vi "Chrg_Dschrg_nodaq_nocrio.vi"(0 "Output Safety":T1, 3 "PS type":enum16{"NHR", "ITECH"}(ring), 4 "PS VISA in":refnum<visa-resource-name>, 5 "PS error in":errorcluster caption="PS error in (no error)", 6 "CyclePath":path=path "C:/Users/ga11/Desktop/VI/results/3PtestCharge.lvm" caption="Filename", 7 "Battery Type":T2(ring), 8 "Charge/discharge":enum8{"Charge", "Discharge"}(ring), 9 "Charge/Discharge Voltage Setpoint":dbl format="%#.6g", 11 "Current Setpoint":dbl format="%#.6g", 13 "Current Cutoff":dbl) -> (14 "PS VISA out":refnum<visa-resource-name>, 19 "PS error out":errorcluster)   [LabVIEW 2020]
uses:
  Drivers-NHR-9200/NHR/Public/Data/Read (Ave Current).vi
  Drivers-NHR-9200/NHR/Public/Data/Low Level/Fetch (Ave Voltage).vi
  Drivers-Essentials/NH Research Regenerative Test Series.lvlib
  Drivers-IT-M3400/IT-M3400.lvlib
panel:
  out "Read Ave Current (A)":dbl
  out "Read Ave Voltage (V)":dbl
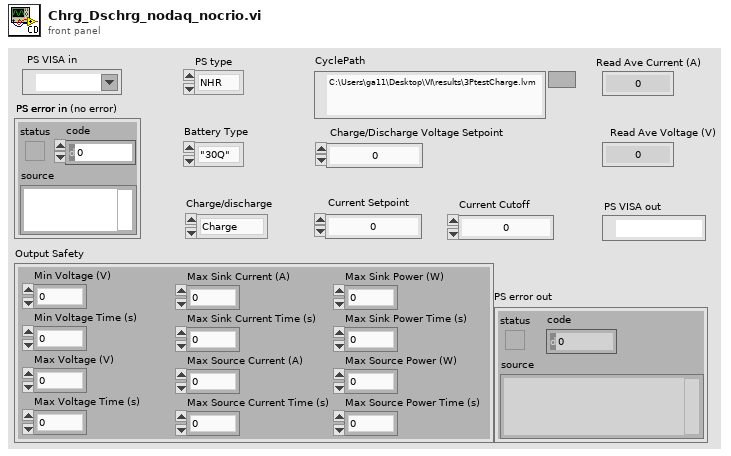
[diagram p1: front panel]
types:
  T1 = cluster{"Min Voltage (V)":dbl, "Min Voltage Time (s)":dbl, "Max Voltage (V)":dbl, "Max Voltage Time (s)":dbl, "Max Sink Current (A)":dbl, "Max Sink Current Time (s)":dbl, "Max Source Current (A)":dbl, "Max Source Current Time (s)":dbl, "Max Sink Power (W)":dbl, "Max Sink Power Time (s)":dbl, "Max Source Power (W)":dbl, "Max Source Power Time (s)":dbl}
  T2 = enum16{"\"30Q\"", "\"40T\"", "\"2P30Q\"", "\"3P30Q\"", "\"Nissan Leaf\""}
  T3 = cluster{"Voltage Enabled":bool, "Current Enabled":bool, "Power Enabled":bool, "Resistance Enabled":bool}
  T4 = cluster{"Baud Rate":u32, "Parity":u16, "Data Bits":u16, "Stop Bits":u16, "Flow Control":u16}
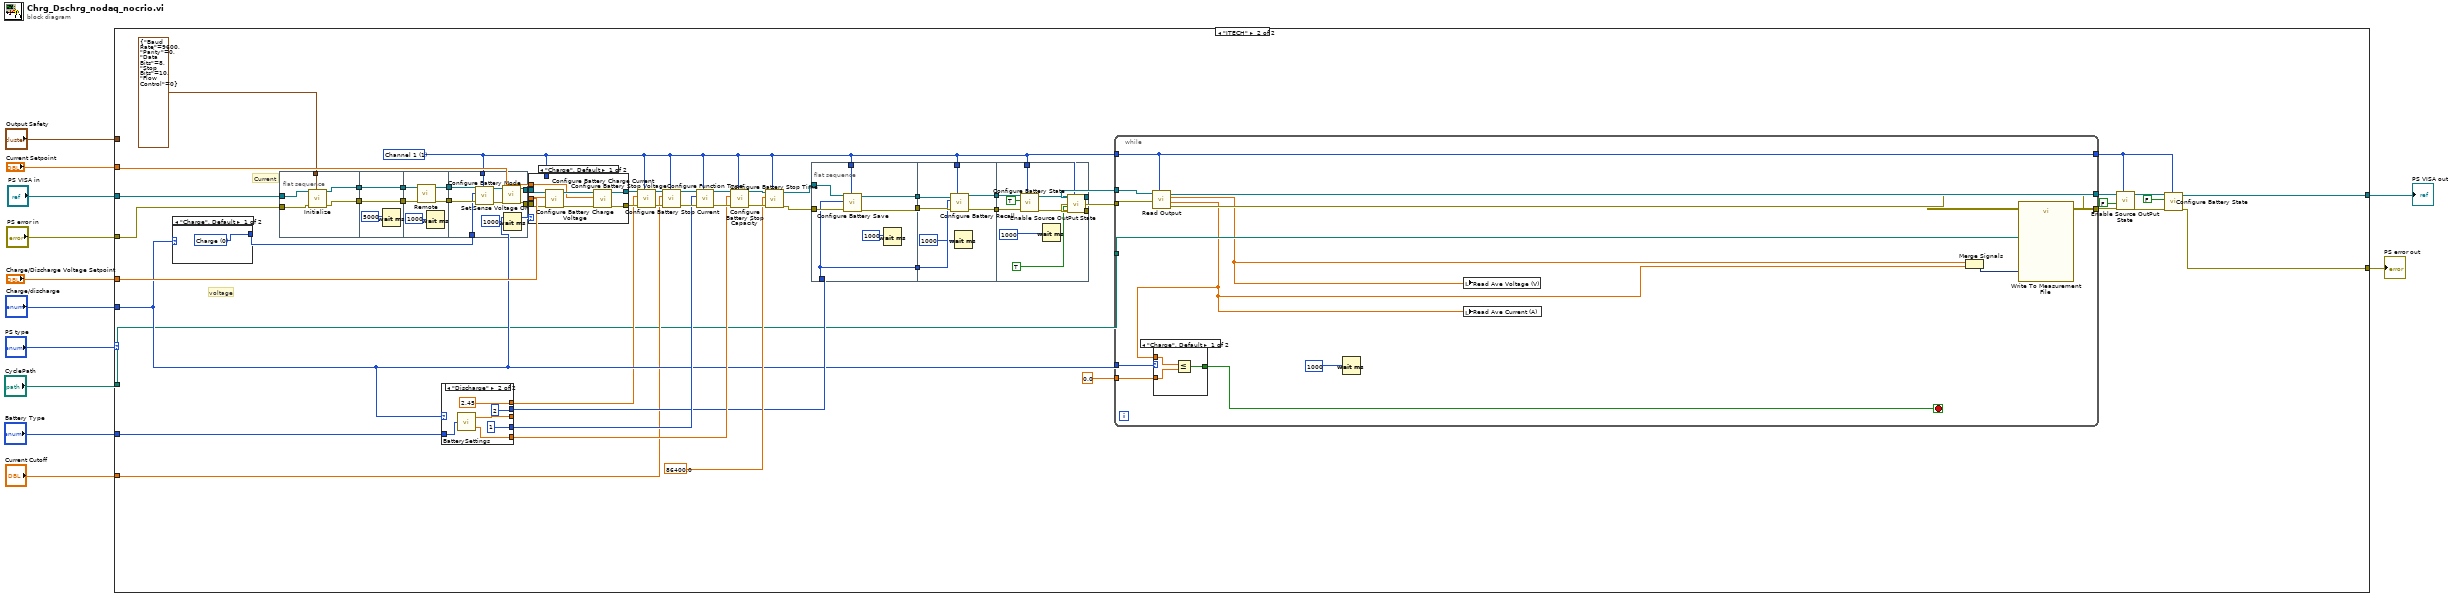
[diagram p0: block diagram]
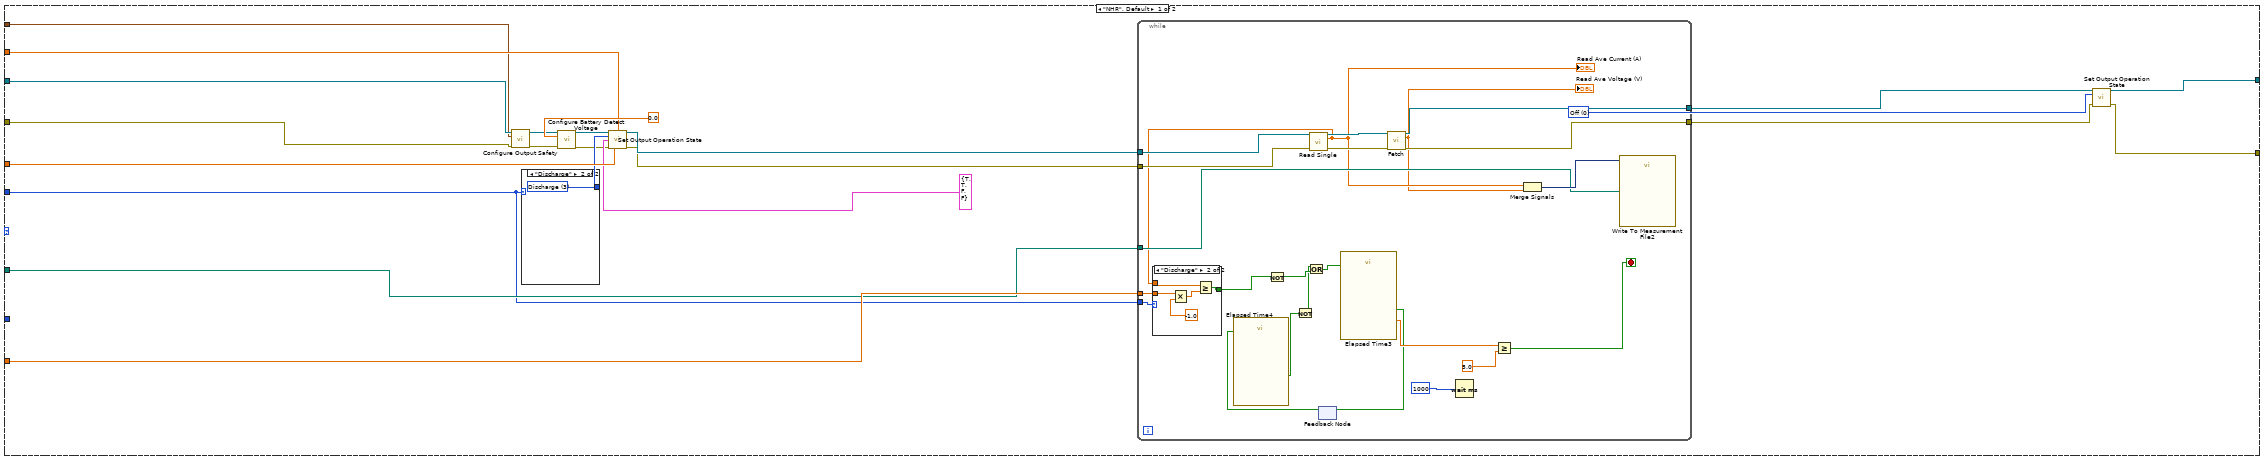
[diagram p2: hidden frame]
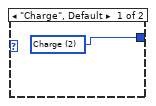
[diagram p3: hidden frame]
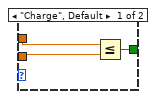
[diagram p4: hidden frame]
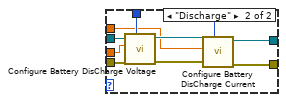
[diagram p5: hidden frame]
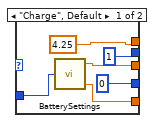
[diagram p6: hidden frame]
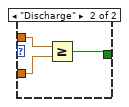
[diagram p7: hidden frame]
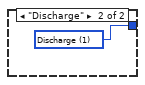
[diagram p8: hidden frame]
diagram:
  n1 = case shown="\"ITECH\"" "PS type" {
    tunnel: "Charge/Discharge Voltage Setpoint" -> [w34 w105]
    tunnel: "Current Setpoint" -> [w18 w103]
    tunnel: "Current Cutoff" -> [w31 w73]
    tunnel: "CyclePath" -> [w28 w71]
    tunnel: "PS VISA in" -> [w14 w84]
    tunnel: "PS error in" -> [w15 w83]
    tunnel: [w23 w70] -> w2
    tunnel: [w22 w104] -> w6
    tunnel: "Charge/discharge" -> [w19 w74]
    tunnel: "Battery Type" -> [_ w102]
    tunnel: "Output Safety" -> [w13 _]
    frame "NHR", Default {
      w27 = 0 items=["Off", "Standby", "Charge", "Discharge", "Battery"] ("Mode (0: Off)")
      n2 = call "Configure Output Safety.vi"("VISA resource name"=w14, "Output Safety"=w13, "error in (no error)"=w15) -> ("VISA resource name out"=w16:refnum<visa-resource-name>, "error out"=w17:errorcluster)  [unwired: 11 in]
      n3 = case shown="\"Discharge\"" w19 {
        tunnel: [w35 w36] -> w29
        frame "Charge", Default {
          w35 = 2 items=["Off", "Standby", "Charge", "Discharge", "Battery"] ("Mode (0: Off)")
        }
        frame "Discharge" {
          w36 = 3 items=["Off", "Standby", "Charge", "Discharge", "Battery"] ("Mode (0: Off)")
        }
      }
      n4 = call "Configure Battery Detect Voltage.vi"("VISA resource name"=w16, "Battery Detect Voltage (0V)"=0.0, "error in (no error)"=w17) -> ("VISA resource name out"=w26:refnum<visa-resource-name>, "error out"=w25:errorcluster)  [unwired: 11 in]
      n5 = call "Set Output Operation State.vi"("VISA resource name"=w26, "Voltage Setpoint (0 V)"=w34, "Current Setpoint (0 A)"=w18, "Mode (0: Off)"=w29, "Enable"=T3 {"Voltage Enabled"=TRUE, "Current Enabled"=TRUE, "Power Enabled"=FALSE, "Resistance Enabled"=FALSE}, "error in (no error)"=w25) -> ("VISA resource name out"=w33:refnum<visa-resource-name>, "error out"=w32:errorcluster)  [unwired: 8 in]
      n6 = while {
        tunnel: w33 -> [w57]
        tunnel: w32 -> [w56]
        tunnel: w31 -> [w41]
        tunnel: w28 -> [w44]
        tunnel: [w43] -> w21
        tunnel: [w42] -> w20
        tunnel: w19 -> [w40]
        stop <- w47 stop-if-true
        n7 = call-poly "Read Single.vi"("VISA resource name"=w57, "error in (no error)"=w56) -> ("VISA resource name out"=w58:refnum<visa-resource-name>, "Ave Current (A)"=w39:dbl, "error out"=w59:errorcluster)  [unwired: 11 in]
        "Read Ave Current (A)" <- w39
        n8 = case shown="\"Discharge\"" w40 {
          tunnel: w41 -> [w61 w66]
          tunnel: w39 -> [w62 w64]
          tunnel: [w60 w63] -> w38
          frame "Charge", Default {
            n9 = Less Or Equal?(x=w62, y=w61) -> (x <= y?=w60:bool)
          }
          frame "Discharge" {
            n10 = Multiply(x=w66, y=-1.0) -> (x*y=w65:dbl)
            n11 = Greater Or Equal?(x=w64, y=w65) -> (x >= y?=w63:bool)
          }
        }
        n12 = Not(x=w38) -> (.not. x?=w53:bool)
        n13 = feedback #1() -> (w45:bool)  [unwired: 1 in]
        n14 = call "Elapsed Time4"("Reset"=w45) -> ("Time has Elapsed"=w52:bool)  [unwired: 11 in, 7 out]
        n15 = Not(x=w52) -> (.not. x?=w51:bool)
        n16 = Or(x=w51, y=w53) -> (x .or. y?=w50:bool)
        n17 = call "Elapsed Time3"("Reset"=w50) -> ("Elapsed Time (s)"=w49:dbl, "Time has Elapsed"=w46:bool)  [unwired: 11 in, 6 out]
        n18 = feedback-in #1(w46) -> ()
        n19 = call-poly "Fetch.vi"("VISA resource name"=w58, "error in (no error)"=w59) -> ("VISA resource name out"=w43:refnum<visa-resource-name>, "Ave Voltage (V)"=w37:dbl, "error out"=w42:errorcluster)  [unwired: 11 in]
        "Read Ave Voltage (V)" <- w37
        n20 = Wait (ms)(milliseconds to wait=1000) -> ()  [unwired: 1 out]
        n21 = Greater Or Equal?(x=w49, y=5.0) -> (x >= y?=w47:bool)
        n22 = Merge Signals "Merge Signals"(w39, w37) -> (w55:dynamicdata)
        n23 = call "Write To Measurement File2"("Signals"=w55, "Filename"=w44) -> ()  [unwired: 15 in, 3 out]
      }
      n24 = call "Set Output Operation State.vi"("VISA resource name"=w21, "Mode (0: Off)"=w27, "error in (no error)"=w20) -> ("VISA resource name out"=w23:refnum<visa-resource-name>, "error out"=w22:errorcluster)  [unwired: 11 in]
    }
    frame "ITECH" {
      w76 = 1 items=["Channel 1"=1, "Channel 2"=2, "Channel 3"=3, "Channel 4"=4, "Channel 5"=5, "Channel 6"=6, "Channel 7"=7, "Channel 8"=8, "Channel 8"=9, "Channel 10"=10, "Channel 11"=11, "Channel 12"=12, "Channel 13"=13, "Channel 14"=14, "Channel 15"=15, "Channel 16"=16] ("Channel")
      # "voltage"
      # "Current"
      n25 = case shown="\"Charge\", Default" w74 {
        tunnel: [w215 w216] -> w90
        frame "Charge", Default {
          w215 = u8 0 items=["Charge", "Discharge"] ("Battery Mode")
        }
        frame "Discharge" {
          w216 = u8 1 items=["Charge", "Discharge"] ("Battery Mode")
        }
      }
      n26 = flat-sequence {
        tunnel: [w121] -> w88
        tunnel: [w122] -> w86
        tunnel: T4 {"Baud Rate"=9600, "Parity"=0, "Data Bits"=8, "Stop Bits"=10, "Flow Control"=0} ("Serial Configuration") -> [w125]
        tunnel: w83 -> [w124]
        tunnel: w84 -> [w123]
        tunnel: w88 -> [w128]
        tunnel: [w128] -> w87
        tunnel: w86 -> [w127]
        tunnel: [w127] -> w85
        tunnel: [w133] -> w92
        tunnel: [w132] -> w91
        tunnel: w87 -> [w131]
        tunnel: w85 -> [w130]
        tunnel: w92 -> [w139]
        tunnel: w91 -> [w141]
        tunnel: w76 -> [w142]
        tunnel: w90 -> [w140]
        tunnel: [w135] -> w69
        tunnel: [w134] -> w68
        frame #0 {
          n27 = call "Initialize.vi"("Serial Configuration"=w125, "error in"=w124, "VISA resource name"=w123) -> ("error out"=w122:errorcluster, "VISA resource name out"=w121:refnum<visa-resource-name>)  [unwired: 7 in]
        }
        frame #1 {
          n28 = Wait (ms)(milliseconds to wait=5000) -> ()  [unwired: 1 out]
        }
        frame #2 {
          n29 = call "Remote.vi"("error in"=w130, "VISA resource name"=w131) -> ("error out"=w132:errorcluster, "VISA resource name out"=w133:refnum<visa-resource-name>)  [unwired: 8 in]
          n30 = Wait (ms)(milliseconds to wait=1000) -> ()  [unwired: 1 out]
        }
        frame #3 {
          n31 = call "Configure Battery Mode.vi"("Channel"=w142, "error in"=w141, "Battery Mode"=w140, "VISA resource name"=w139) -> ("error out"=w136:errorcluster, "VISA resource name out"=w137:refnum<visa-resource-name>)  [unwired: 6 in]
          n32 = call "Set Sense Voltage On.vi"("error in"=w136, "VISA resource name"=w137) -> ("error out"=w135:errorcluster, "VISA resource name out"=w134:refnum<visa-resource-name>)  [unwired: 8 in]
          n33 = Wait (ms)(milliseconds to wait=1000) -> ()  [unwired: 1 out]
        }
      }
      n34 = case shown="\"Discharge\"" w74 {
        tunnel: w102 -> [w189 w195]
        tunnel: [w188 w193] -> _
        tunnel: [u8 0 ("File") u8 1 ("File")] -> w78
        tunnel: [u8 1 ("File") u8 2 ("File")] -> w75
        tunnel: [w185 w191] -> w77
        tunnel: [4.25 2.45] -> w72
        frame "Charge", Default {
          n35 = call "BatterySettings.vi"("Battery Type"=w189) -> ("RatedCapacity (Ah)"=w185:dbl, "Max Voltage (V)"=w188:dbl)  [unwired: 2 in, 1 out]
        }
        frame "Discharge" {
          n36 = call "BatterySettings.vi"("Battery Type"=w195) -> ("RatedCapacity (Ah)"=w191:dbl, "Min Voltage (V)"=w193:dbl)  [unwired: 2 in, 1 out]
        }
      }
      n37 = case shown="\"Charge\", Default" w74 {
        tunnel: w68 -> [w174 w183]
        tunnel: w69 -> [w173 w182]
        tunnel: [w168 w179] -> w112
        tunnel: [w167 w178] -> w111
        tunnel: w76 -> [_ w177]
        tunnel: w105 -> [w170 w176]
        tunnel: w103 -> [w169 w175]
        frame "Charge", Default {
          n38 = call "Configure Battery Charge Voltage.vi"("error in"=w173, "Charge Voltage(V)"=w170, "VISA resource name"=w174) -> ("error out"=w171:errorcluster, "VISA resource name out"=w172:refnum<visa-resource-name>)  [unwired: 6 in]
          n39 = call "Configure Battery Charge Current.vi"("error in"=w171, "Charge Current(A)"=w169, "VISA resource name"=w172) -> ("error out"=w167:errorcluster, "VISA resource name out"=w168:refnum<visa-resource-name>)  [unwired: 7 in]
        }
        frame "Discharge" {
          n40 = call "Configure Battery DisCharge Voltage.vi"("Channel"=w177, "error in"=w182, "Discharge Voltage(V)"=w176, "VISA resource name"=w183) -> ("error out"=w180:errorcluster, "VISA resource name out"=w181:refnum<visa-resource-name>)  [unwired: 6 in]
          n41 = call "Configure Battery DisCharge Current.vi"("Channel"=w177, "error in"=w180, "Discharge Current(A)"=w175, "VISA resource name"=w181) -> ("error out"=w178:errorcluster, "VISA resource name out"=w179:refnum<visa-resource-name>)  [unwired: 6 in]
        }
      }
      n42 = call "Configure Battery Stop Voltage.vi"("Channel"=w76, "error in"=w111, "Stop Voltage(V)"=w72, "VISA resource name"=w112) -> ("error out"=w119:errorcluster, "VISA resource name out"=w120:refnum<visa-resource-name>)  [unwired: 6 in]
      n43 = call "Configure Battery Stop Current.vi"("Channel"=w76, "error in"=w119, "Stop Current(A)"=w73, "VISA resource name"=w120) -> ("error out"=w80:errorcluster, "VISA resource name out"=w82:refnum<visa-resource-name>)  [unwired: 6 in]
      n44 = call "Configure Function Type.vi"("Channel"=w76, "error in"=w80, "Function Type"=w78, "VISA resource name"=w82) -> ("error out"=w79:errorcluster, "VISA resource name out"=w81:refnum<visa-resource-name>)  [unwired: 6 in]
      n45 = call "Configure Battery Stop Capacity.vi"("Channel"=w76, "error in"=w79, "Stop Capacity(Ah)"=w77, "VISA resource name"=w81) -> ("error out"=w117:errorcluster, "VISA resource name out"=w118:refnum<visa-resource-name>)  [unwired: 6 in]
      n46 = call "Configure Battery Stop Time.vi"("Channel"=w76, "error in"=w117, "Stop Time(S)"=86400.0, "VISA resource name"=w118) -> ("error out"=w94:errorcluster, "VISA resource name out"=w93:refnum<visa-resource-name>)  [unwired: 6 in]
      n47 = flat-sequence {
        tunnel: w75 -> [w148]
        tunnel: w76 -> [w143]
        tunnel: [w146] -> w97
        tunnel: [w148] -> w96
        tunnel: [w145] -> w95
        tunnel: w94 -> [w149]
        tunnel: w93 -> [w147]
        tunnel: [w152] -> w99
        tunnel: [w153] -> w98
        tunnel: w97 -> [w156]
        tunnel: w96 -> [w155]
        tunnel: w95 -> [w154]
        tunnel: w76 -> [w150]
        tunnel: [w160] -> w110
        tunnel: [w159] -> w109
        tunnel: w76 -> [w158]
        tunnel: w99 -> [w166]
        tunnel: w98 -> [w165]
        frame #0 {
          n48 = call "Configure Battery Save.vi"("Channel"=w143, "error in"=w149, "File"=w148, "VISA resource name"=w147) -> ("error out"=w146:errorcluster, "VISA resource name out"=w145:refnum<visa-resource-name>)  [unwired: 6 in]
          n49 = Wait (ms)(milliseconds to wait=1000) -> ()  [unwired: 1 out]
        }
        frame #1 {
          n50 = call "Configure Battery Recall.vi"("Channel"=w150, "error in"=w156, "File"=w155, "VISA resource name"=w154) -> ("error out"=w153:errorcluster, "VISA resource name out"=w152:refnum<visa-resource-name>)  [unwired: 6 in]
          n51 = Wait (ms)(milliseconds to wait=1000) -> ()  [unwired: 1 out]
        }
        frame #2 {
          n52 = call "Configure Battery State.vi"("Channel"=w158, "error in"=w165, "State"=TRUE, "VISA resource name"=w166) -> ("error out"=w163:errorcluster, "VISA resource name out"=w164:refnum<visa-resource-name>)  [unwired: 6 in]
          n53 = Wait (ms)(milliseconds to wait=1000) -> ()  [unwired: 1 out]
          n54 = call "Enable Source OutPut State.vi"("Channel"=w158, "error in"=w163, "State"=TRUE ("Enable Output|Intput"), "VISA resource name"=w164) -> ("error out"=w159:errorcluster, "VISA resource name out"=w160:refnum<visa-resource-name>)  [unwired: 6 in]
        }
      }
      n55 = while {
        tunnel: [w200] -> w108
        tunnel: [w198] -> w107
        tunnel: w110 -> [w208]
        tunnel: w109 -> [w207]
        tunnel: w76 -> [w199]
        tunnel: [w199] -> w106
        tunnel: w71 -> [w205]
        tunnel: 0.0 -> [w203]
        tunnel: w74 -> [w201]
        stop <- w202 stop-if-true
        n56 = call "Read Output.vi"("Channel"=w199, "error in"=w207, "VISA resource name"=w208) -> ("error out"=w198:errorcluster, "Read Current(A)"=w196:dbl, "Read Voltage(V)"=w197:dbl, "VISA resource name out"=w200:refnum<visa-resource-name>)  [unwired: 5 in]
        n57 = case shown="\"Charge\", Default" w201 {
          tunnel: w203 -> [w210 w213]
          tunnel: w196 -> [w211 w214]
          tunnel: [w209 w212] -> w202
          frame "Charge", Default {
            n58 = Less Or Equal?(x=w211, y=w210) -> (x <= y?=w209:bool)
          }
          frame "Discharge" {
            n59 = Greater Or Equal?(x=w214, y=w213) -> (x >= y?=w212:bool)
          }
        }
        n60 = Wait (ms)(milliseconds to wait=1000) -> ()  [unwired: 1 out]
        n61 = local write "Read Ave Voltage (V)"(w197) -> ()
        n62 = local write "Read Ave Current (A)"(w196) -> ()
        n63 = Merge Signals "Merge Signals"(w197, w196) -> (w206:dynamicdata)
        n64 = call "Write To Measurement File"("Signals"=w206, "Filename"=w205) -> ()  [unwired: 15 in, 3 out]
      }
      n65 = call "Enable Source OutPut State.vi"("Channel"=w106, "error in"=w107, "State"=FALSE, "VISA resource name"=w108) -> ("error out"=w115:errorcluster, "VISA resource name out"=w116:refnum<visa-resource-name>)  [unwired: 6 in]
      n66 = call "Configure Battery State.vi"("Channel"=w106, "error in"=w115, "State"=FALSE, "VISA resource name"=w116) -> ("error out"=w104:errorcluster, "VISA resource name out"=w70:refnum<visa-resource-name>)  [unwired: 6 in]
    }
  }
  "PS error out" <- w6
  "PS VISA out" <- w2
